vi "Open References To All Libraries And VIs In Project.vi"(8 "error in (no error)":errorcluster, 9 "Exclude Targets? (F)":bool, 10 "Exclude Dependencies? (T)":bool=TRUE, 11 "Project in":refnum<vi>) -> (0 "error out":errorcluster, 2 "VI and Library References":T1[](array[typedef]), 3 "Project out":refnum<vi>)   [LabVIEW 2017, in "Edit LVProj.lvlib"]
uses:
  <vilib>/Utility/EditLVProj/Edit LVProj.lvlib
  <vilib>/Utility/EditLVProj/Library And VI References.ctl
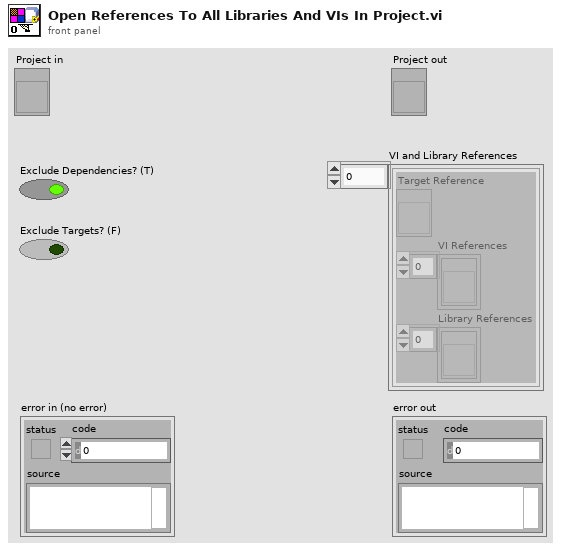
[diagram p1: front panel]
types:
  T1 = typedef "Edit LVProj.lvlib/Library And VI References.ctl" = cluster{"Target Reference":refnum<vi>, "VI References":refnum<vi>[], "Library References":refnum<vi>[]}
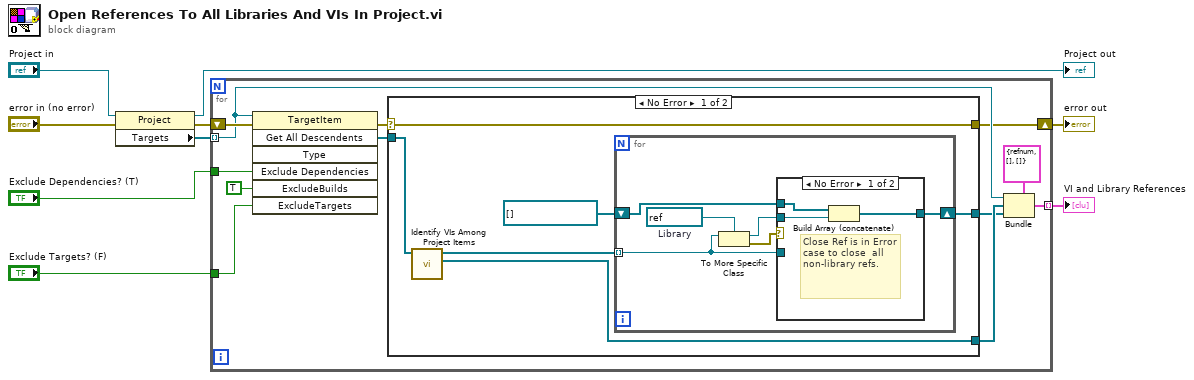
[diagram p0: block diagram]
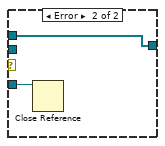
[diagram p2: hidden frame]
diagram:
  n1 = property class="Project"(reference="Project in", error in="error in (no error)") -> (reference out=→"Project out":refnum<vi>, error out=w6:errorcluster, "Targets"=w4:refnum<vi>[])
  n2 = for {
    tunnel: "Exclude Dependencies? (T)" -> [w19]
    tunnel: w4 -> [w15] mode=indexing
    tunnel: [w16] -> w3 mode=indexing
    shift-right: [w13] -> w2
    shift-left: w6 -> [w20]
    tunnel: "Exclude Targets? (F)" -> [w10]
    n3 = invoke class="TargetItem" method="Get All Descendents"(reference=w15, error in=w20, "Exclude Dependencies"=w19, "ExcludeBuilds"=TRUE, "ExcludeTargets"=w10) -> (error out=w11:errorcluster, "All Descendents"=w21:refnum<vi>[])  [unwired: 2 in, 5 out]
    n4 = case shown="No Error" w11 {
      selector: w11 -> [w22 w39]
      tunnel: w21 -> [w26 _]
      tunnel: [w24 _] -> w18
      tunnel: [w23 _] -> w17
      tunnel: [w22 w39] -> w13
      frame No Error {
        n5 = call <vilib>:"Identify VIs Among Project Items.vi"("Project Item References in"=w26) -> ("VI References"=w24:refnum<vi>[], "Project Item References out"=w25:refnum<vi>[])  [unwired: 9 in]
        n6 = for {
          tunnel: w25 -> [w30] mode=indexing
          shift-right: [w28] -> w23
          shift-left: refnum<vi>[] [] -> [w29]
          w33 = refnum<vi> refnum  # Library
          n7 = To More Specific Class(target class=w33, reference=w30) -> (specific class reference=w32:refnum<vi>, error out=w31:errorcluster)  [unwired: 1 in]
          n8 = case shown="No Error" w31 {
            tunnel: w32 -> [w35 _]
            tunnel: w30 -> [_ w38]
            tunnel: w29 -> [w36 w37]
            tunnel: [w34 w37] -> w28
            frame No Error {
              # "Close Ref is in Error case to close  all non-library refs."
              n9 = Build Array (concatenate)(w36, w35) -> (w34:refnum<vi>[])
            }
            frame Error {
              n10 = Close Reference(reference=w38) -> ()  [unwired: 1 in, 1 out]
            }
          }
        }
      }
      frame Error {
      }
    }
    n11 = Bundle(cluster=T1 {"Target Reference"=refnum, "VI References"=[], "Library References"=[]} ("Edit LVProj.lvlib:Library And VI References"), "Target Reference"=w15, "VI References"=w18, "Library References"=w17) -> (w16:T1)
  }
  "error out" <- w2
  "VI and Library References" <- w3
